vi "CanControlInitialize.vi"(4 "Operating Mode":T1, 5 "error in":errorcluster {"code" format="%.0x"}, 6 "BTR 0":u8 format="%02x", 7 "BTR 1":u8 format="%02x", 8 "CAN Control Handle in":u32 format="%x") -> (0 "error out":errorcluster {"code" format="%.0x"}, 2 "InitOK":bool, 3 "CAN Control Handle out":u32)   [LabVIEW 2011]
doc: "Initializes the CAN controller in the specified operating mode and bit rate."
uses:
  vcilva.dll
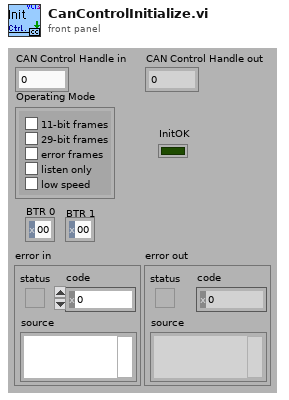
[diagram p1: front panel]
types:
  T1 = cluster{"standard":bool, "extended":bool, "errorframes":bool, "listenonly":bool, "lowspeed":bool}
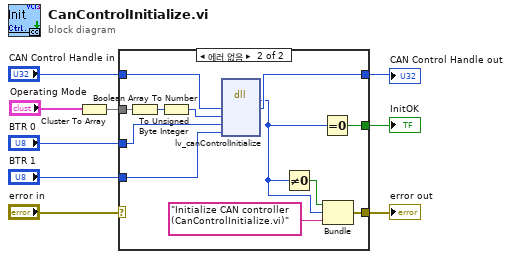
[diagram p0: block diagram]
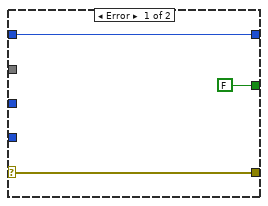
[diagram p2: hidden frame]
diagram:
  n1 = Cluster To Array(cluster="Operating Mode") -> (array=w3:bool[])
  n2 = case shown="에러 없음" "error in" {
    selector: "error in" -> [w12 _]
    tunnel: [w12 w24] -> w8
    tunnel: "CAN Control Handle in" -> [w11 w21]
    tunnel: [w11 w20] -> w6
    tunnel: "BTR 0" -> [_ w19]
    tunnel: "BTR 1" -> [_ w18]
    tunnel: w3 -> [_ w15]
    tunnel: [FALSE w14] -> w1
    frame Error {
    }
    frame No Error {
      n3 = Boolean Array To Number(Boolean array=w15) -> (number=w16:u32)
      n4 = To Unsigned Byte Integer(number=w16) -> (unsigned 8bit integer=w17:u8)
      n5 = dll-call lib="vcilva.dll" fn="lv_canControlInitialize"("hCanCtl"=w21, "bMode"=w17, "bBtr0"=w19, "bBtr1"=w18) -> (w13:i32, "hCanCtl"=w20:u32)  [unwired: 6 in, 2 out]
      n6 = Not Equal To 0?(x=w13) -> (x != 0?=w23:bool)
      n7 = Equal To 0?(x=w13) -> (x = 0?=w14:bool)
      n8 = Bundle(w23, w13, "Initialize CAN controller (CanControlInitialize.vi)") -> (w24:errorcluster)  [unwired: 1 in]
    }
  }
  "error out" <- w8
  "CAN Control Handle out" <- w6
  "InitOK" <- w1
